vi "Edit Tag Window.vi"(7 "Database Connection":refnum<k7>, 8 "Error In":errorcluster, 11 "TagId":string) -> (0 "Error Out":errorcluster)   [LabVIEW 2019]
uses:
  Controls/Tag Settings.ctl
panel:
  in  "TagData":T1 {"Vmax" min=-10.0 max=10.0 step=1.0; "Vmin" min=-10.0 max=10.0 step=1.0}
  in  "Cancel Button":bool
  in  "OK Button":bool
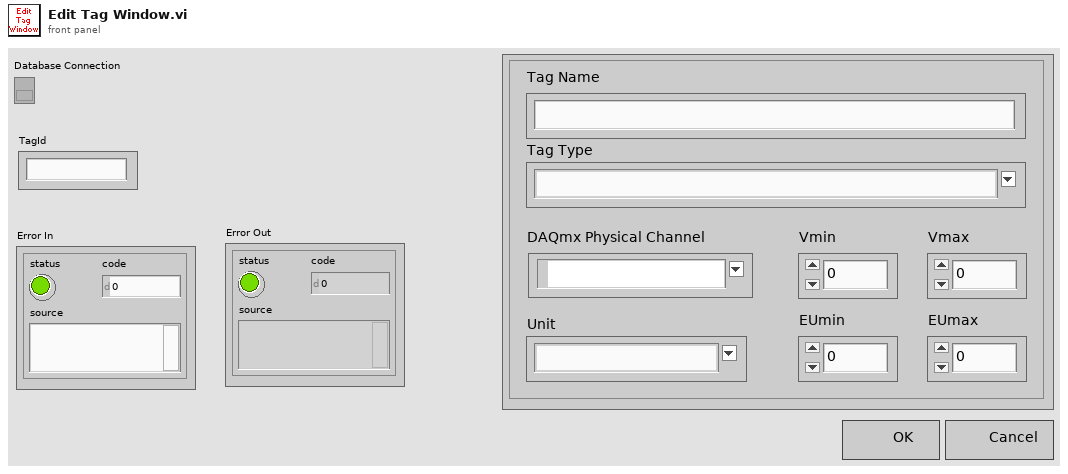
[diagram p1: front panel]
types:
  T1 = typedef "Tag Settings.ctl" = cluster{"Tag Name":string, "Tag Type":string, "DAQmx Physical Channel":tag, "Vmin":dbl, "Vmax":dbl, "Unit":string, "EUmin":dbl, "EUmax":dbl}
  T2 = typedef "Device Settings.ctl" = cluster{"Device Type":string, "Device Name":string, "DAQmx Name":tag, "Terminal Wiring":i32}
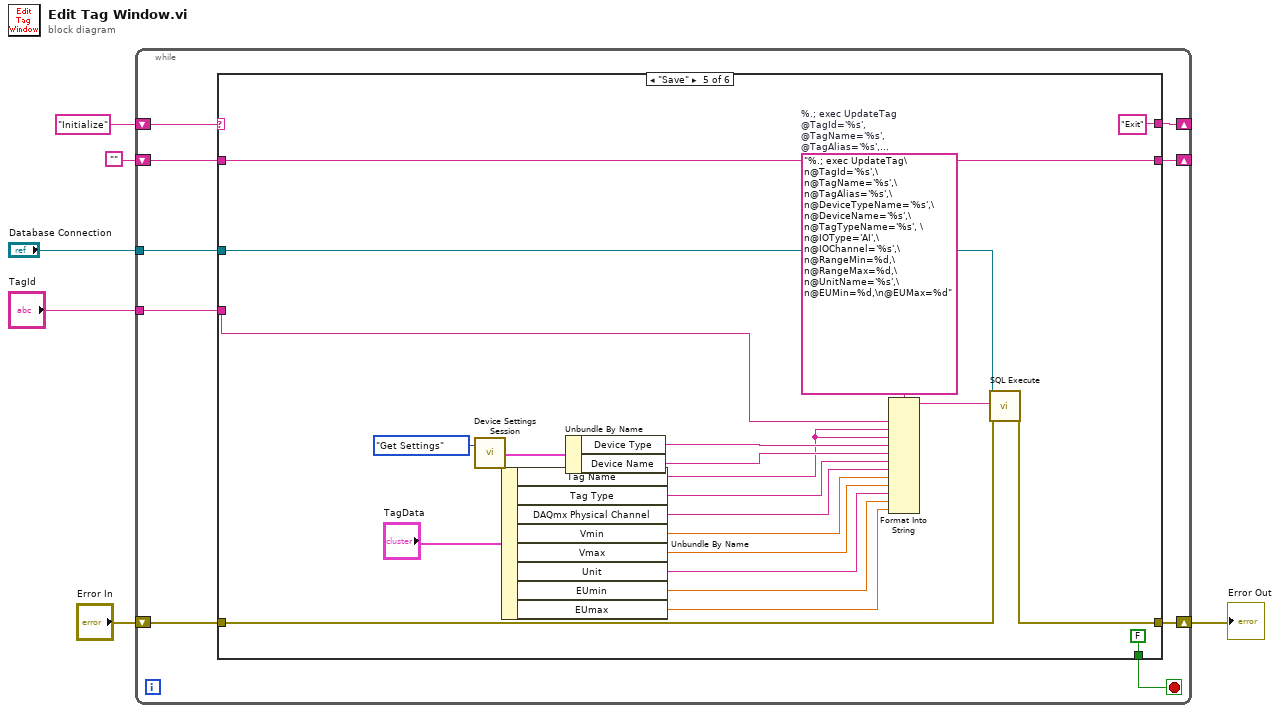
[diagram p0: block diagram]
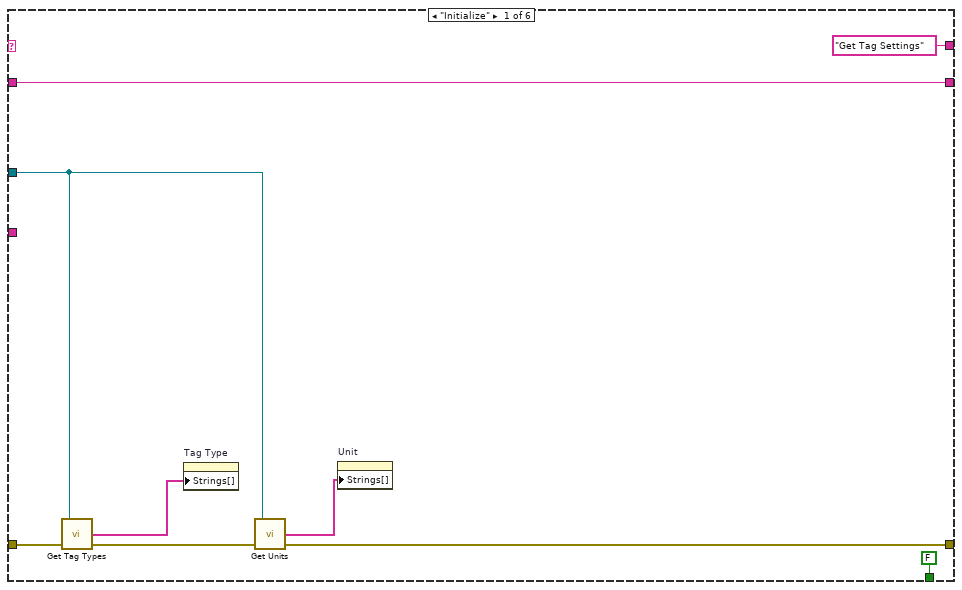
[diagram p2: hidden frame]
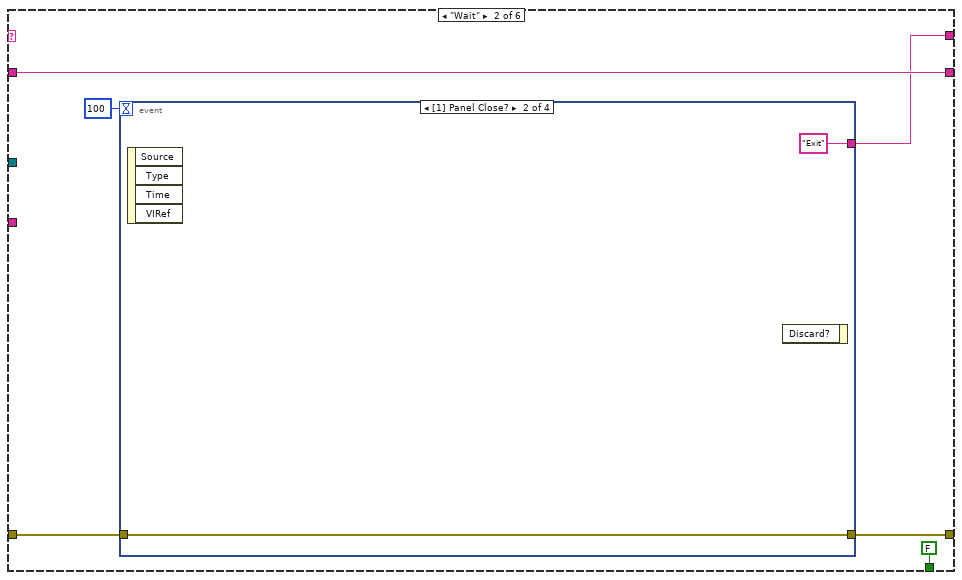
[diagram p3: hidden frame]
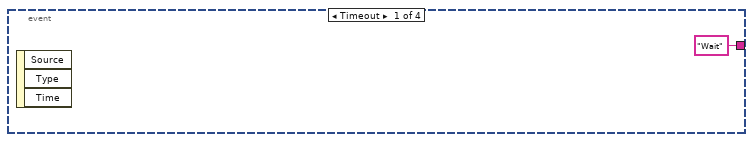
[diagram p4: hidden frame]
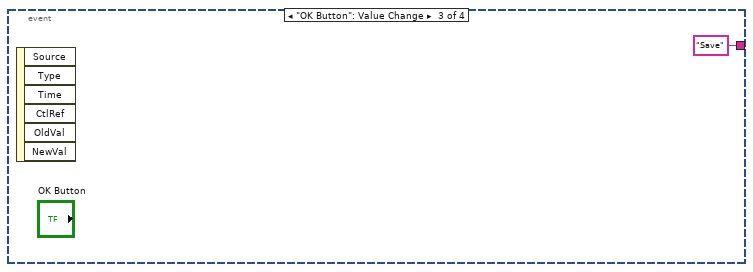
[diagram p5: hidden frame]
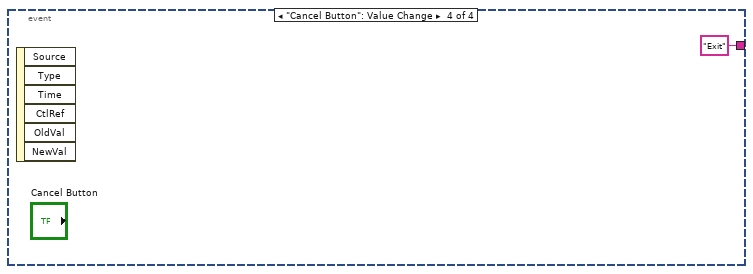
[diagram p6: hidden frame]
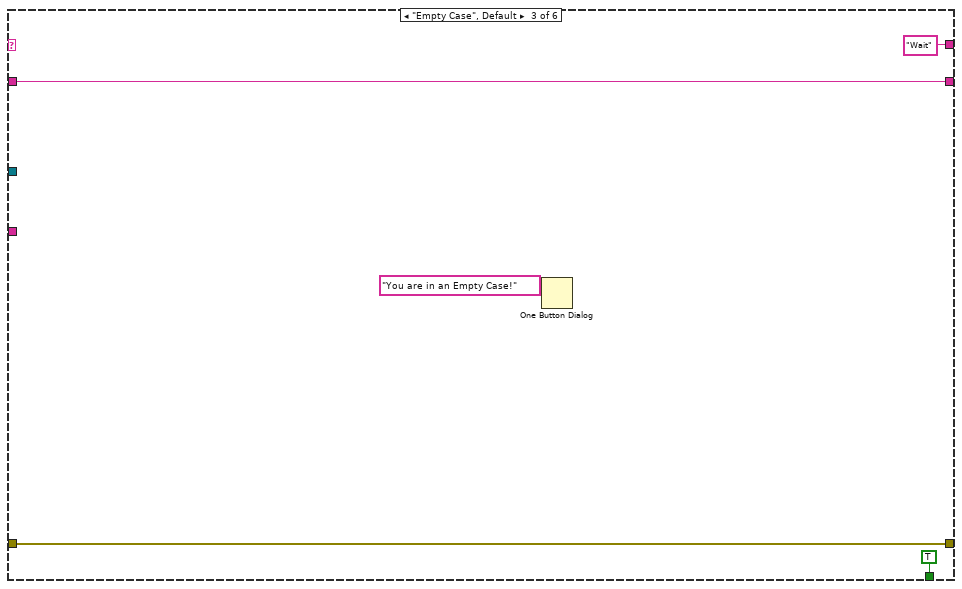
[diagram p7: hidden frame]
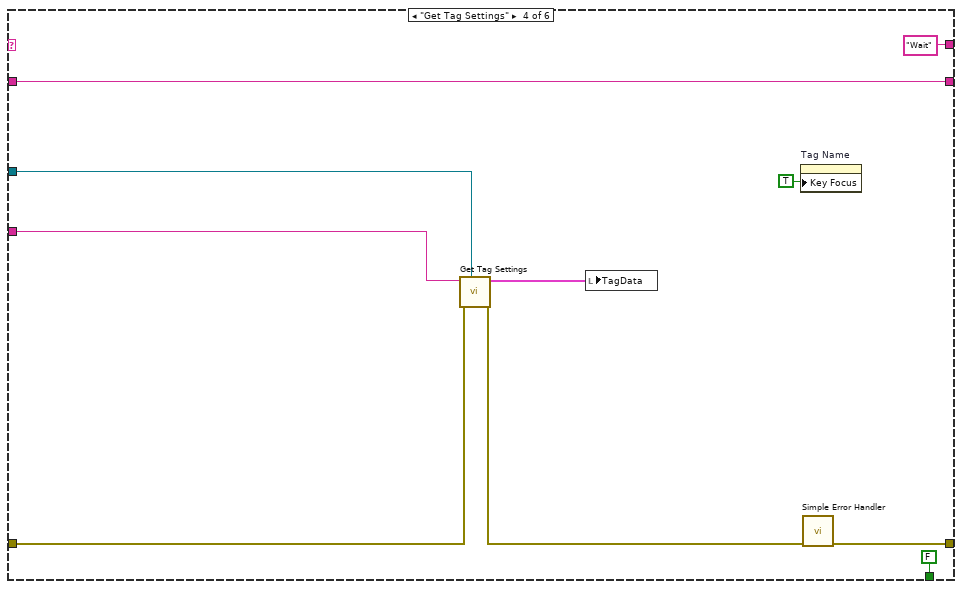
[diagram p8: hidden frame]
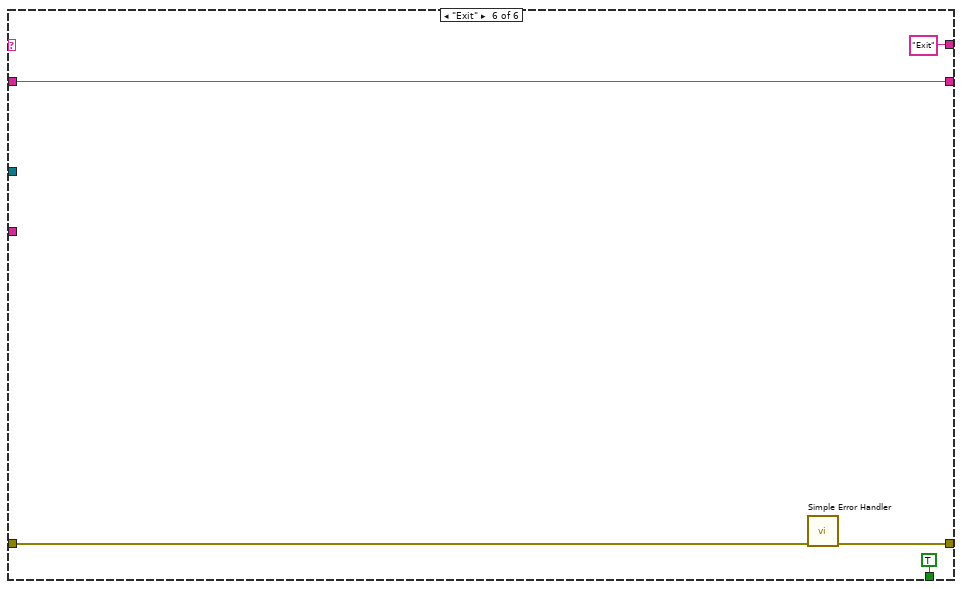
[diagram p9: hidden frame]
diagram:
  n1 = while {
    shift-right: [w11] -> _
    shift-left: "Initialize" ("key") -> [w15]
    shift-right: [w12] -> _
    shift-left: "" -> [w14]
    shift-right: [w9] -> w4
    shift-left: "Error In" -> [w13]
    tunnel: "Database Connection" -> [w8]
    tunnel: "TagId" -> [w7]
    stop <- w10 stop-if-true
    n2 = case shown="\"Save\"" w15 {
      tunnel: w14 -> [w22 w29 w37 w48 w70 w77]
      tunnel: w13 -> [w17 w26 w38 w46 w55 w74]
      tunnel: [w22 w29 w37 w48 w70 w77] -> w12
      tunnel: ["Get Tag Settings" ("key") w28 "Wait" ("key") "Wait" ("key") "Exit" ("key") "Exit" ("key")] -> w11
      tunnel: [FALSE FALSE TRUE FALSE FALSE TRUE] -> w10
      tunnel: [w16 w25 w38 w42 w54 w73] -> w9
      tunnel: w8 -> [w18 _ _ w44 w51 _]
      tunnel: w7 -> [_ _ _ w45 w52 _]
      frame "Initialize" {
        n3 = call "Get Tag Types.vi"("Error In"=w17, "Database Connection"=w18) -> ("Error Out"=w20:errorcluster, "TagTypeNames"=w19:string[])  [unwired: 1 in, 1 out]
        n4 = property on="Tag Type" class="CmbBox"("Strings[]"=w19) -> ()  [unwired: 2 in, 2 out]
        n5 = call "Get Units.vi"("Error In"=w20, "Database Connection"=w18) -> ("Error Out"=w16:errorcluster, "UnitNames"=w21:string[])  [unwired: 1 in, 1 out]
        n6 = property on="Unit" class="CmbBox"("Strings[]"=w21) -> ()  [unwired: 2 in, 2 out]
      }
      frame "Wait" {
        n7 = event shown="[1] Panel Close?" {
          selector: _ -> [_ _ _ _]
          dyn-events: _ -> [_ _ _ _]
          timeout: 100 -> [_ _ _ _]
          tunnel: ["Wait" ("key") "Exit" ("key") "Save" ("key") "Exit" ("key")] -> w28
          tunnel: w26 -> [_ w32 _ _]
          tunnel: [_ w32 _ _] -> w25
          event Timeout {
            n8 = event-data() -> ()  [unwired: 1 in, 3 out]
          }
          event Panel Close? {
            n9 = event-data() -> ()  [unwired: 1 in, 4 out]
            n10 = event-data() -> ()  [unwired: 2 in, 1 out]
          }
          event "OK Button": Value Change {
            n11 = event-data() -> ()  [unwired: 1 in, 6 out]
          }
          event "Cancel Button": Value Change {
            n12 = event-data() -> ()  [unwired: 1 in, 6 out]
          }
        }
      }
      frame "Empty Case", Default {
        n13 = One Button Dialog(message="You are in an Empty Case!") -> ()  [unwired: 1 in, 1 out]
      }
      frame "Get Tag Settings" {
        n14 = call "Get Tag Settings.vi"("Database Connection"=w44, "Error In"=w46, "TagId"=w45) -> ("Error Out"=w43:errorcluster, "TagData"=w47:T1)  [unwired: 7 in]
        n15 = local write "TagData"(w47) -> ()
        n16 = property on="Tag Name" class="Str"("Key Focus"=TRUE) -> ()  [unwired: 2 in, 2 out]
        n17 = call <vilib>:"Simple Error Handler.vi"("error in (no error)"=w43) -> ("error out"=w42:errorcluster)  [unwired: 4 in, 4 out]
      }
      frame "Save" {
        w69 = "%.; exec UpdateTag\n@TagId='%s',\n@TagName='%s',\n@TagAlias='%s',\n@DeviceTypeName='%s',\n@DeviceName='%s',\n@TagTypeName='%s', \n@IOType='AI',\n@IOChannel='%s',\n@RangeMin=%d,\n@RangeMax=%d,\n@UnitName='%s',\n@EUMin=%d,\n@EUMax=%d"  # %.; exec UpdateTag @TagId='%s', @TagName='%s', @TagAlias='%s', @DeviceTypeName='%s', @DeviceName='%s', @TagTypeName='%s',  @IOType='AI', @IOChannel='%s', @RangeMin=%d, @RangeMax=%d, @UnitName='%s', @EUMin=%d, @EUMax=%d
        n18 = call "Device Settings Session.vi"("Type"=enum16{"Set Settings", "Get Settings"}."Get Settings") -> ("Device Settings"=w67:T2)  [unwired: 1 in, 1 out]
        n19 = Unbundle By Name("TagData") -> ("Tag Name"=w53:string, "Tag Type"=w64:string, "DAQmx Physical Channel"=w63:tag, "Vmin"=w62:dbl, "Vmax"=w61:dbl, "Unit"=w60:string, "EUmin"=w59:dbl, "EUmax"=w58:dbl)
        n20 = Unbundle By Name(w67) -> ("Device Type"=w66:string, "Device Name"=w65:string)
        n21 = Format Into String(format string=w69, w52, w53, w53, w66, w65, w64, w63, w62, w61, w60, w59, w58) -> (resulting string=w68:string)  [unwired: 2 in, 1 out]
        n22 = call <vilib>:"SQL Execute.vi"("Connection In"=w51, "SQL Query"=w68, "Error in (no error)"=w55) -> ("Error out"=w54:errorcluster)  [unwired: 15 in, 1 out]
      }
      frame "Exit" {
        n23 = call <vilib>:"Simple Error Handler.vi"("error in (no error)"=w74) -> ("error out"=w73:errorcluster)  [unwired: 4 in, 4 out]
      }
    }
  }
  "Error Out" <- w4
